vi "MSEncoder SubVI DynamicTimeout_Reset.vi"(8 "error in (no error)":errorcluster, 11 "MSEncoder in":refnum<class "MSEncoder.lvclass">) -> (0 "error out":errorcluster, 3 "MSEncoder out":refnum<class "MSEncoder.lvclass">)   [LabVIEW 2018, in "MSEncoder.lvclass"]
uses:
  MSEncoder.lvclass
  MSEncoder.lvclass/MSEncoder.ctl
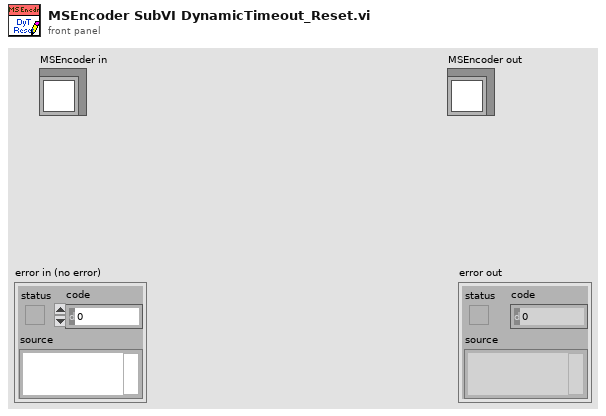
[diagram p1: front panel]
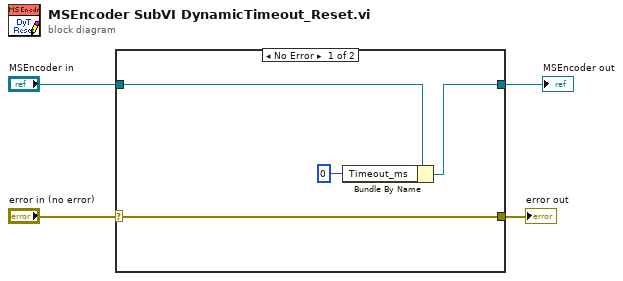
[diagram p0: block diagram]
diagram:
  n1 = case shown="No Error" "error in (no error)" {
    selector: "error in (no error)" -> [w8 w9]
    tunnel: [w8 w9] -> w3
    tunnel: [w7 w10] -> w2
    tunnel: "MSEncoder in" -> [w6 w10]
    frame No Error {
      n2 = Bundle By Name(cluster=w6, "Timeout_ms"=0) -> (w7:refnum<class "MSEncoder.lvclass">)
    }
    frame Error {
    }
  }
  "error out" <- w3
  "MSEncoder out" <- w2
